vi "SerialComMain.vi"() -> ()   [LabVIEW 2021]
uses:
  MainDataTypedef.ctl
  <vilib>/Instr/_visa.llb/VISA Configure Serial Port (Instr).vi
panel:
  out "bytes read":u32
  out "NowTime":timestamp
  in  "ClosePort":bool
  in  "OpenProt":bool
  in  "flow control":u16(ring) items=["None"=0, "XON/XOFF"=1, "RTS/CTS"=2, "DTR/DSR"=4]
  in  "stop bits":u16(ring)=10 items=["1.0"=10, "1.5"=15, "2.0"=20]
  in  "parity":u16(ring) items=["None", "Odd", "Even", "Mark", "Space"]
  in  "data bits":u16=8 min=5 max=8 step=1
  in  "baud rate":u32=9600
  in  "delay before read (ms)":u32=500
  in  "VISA resource name":refnum<visa-resource-name>="COM1"
  out "Response":string
  in  "Command":string="*IDN?\n"
  in  "SerialSend":bool
  out "MsgString":string
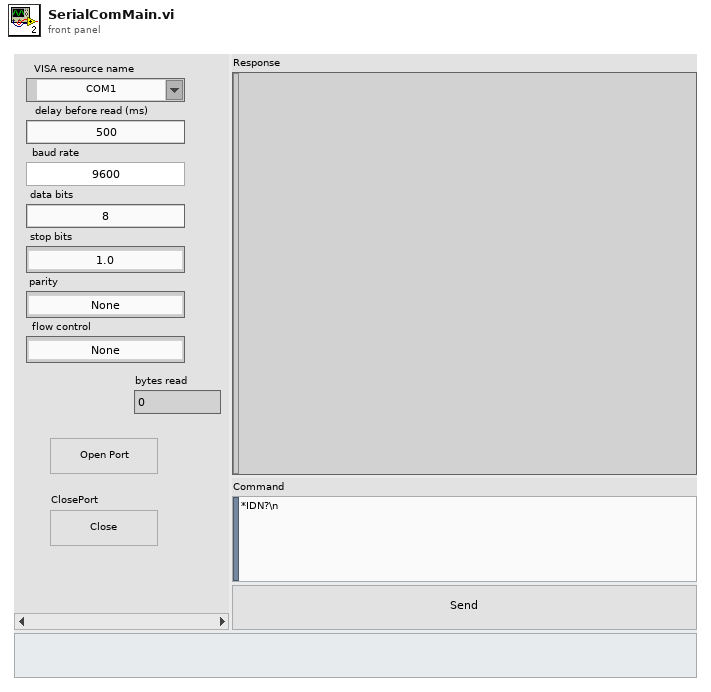
[diagram p1: front panel]
types:
  T1 = typedef "MainDataTypedef.ctl" = cluster{"NowTime":timestamp, "MsgString":string, "VISAResource":refnum<visa-resource-name>, "BytesRead":u32, "Respones":string, "PortOpen?":bool}
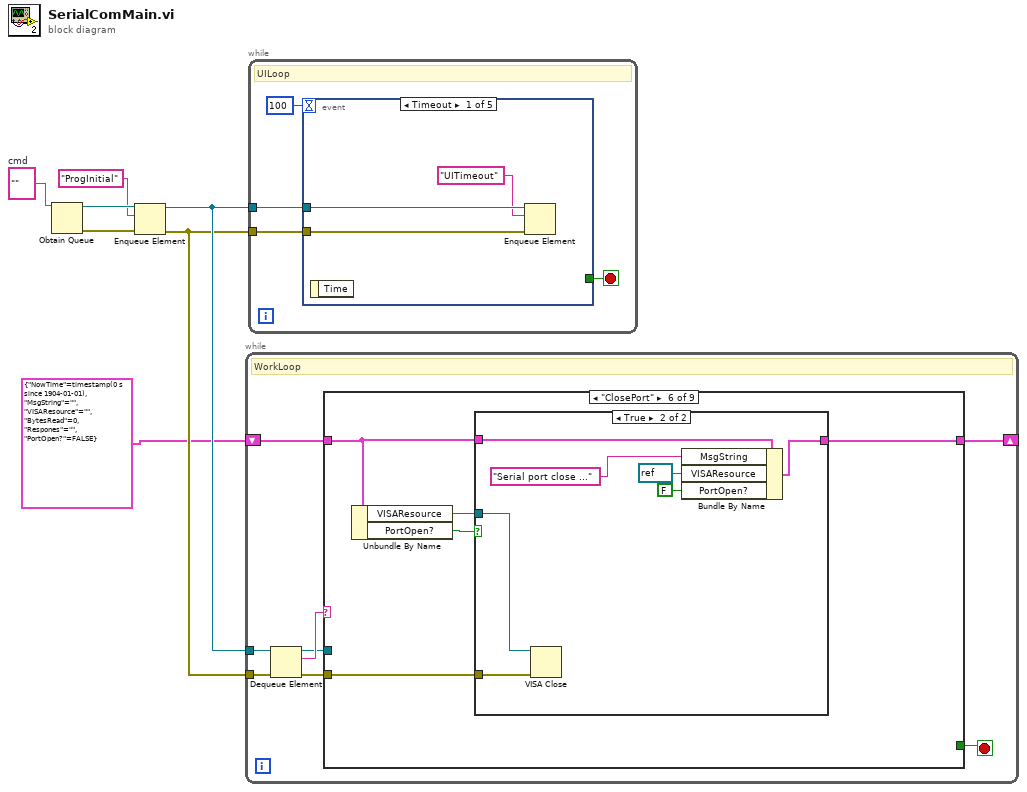
[diagram p0: block diagram]
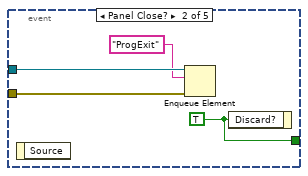
[diagram p2: hidden frame]
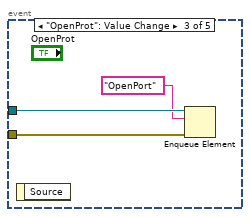
[diagram p3: hidden frame]
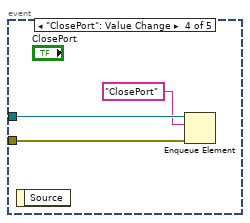
[diagram p4: hidden frame]
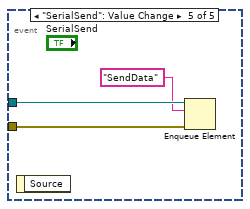
[diagram p5: hidden frame]
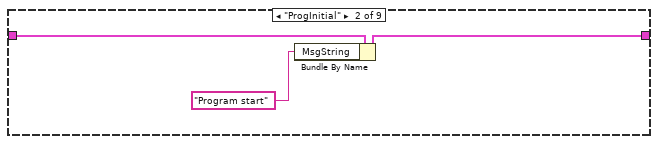
[diagram p7: hidden frame]
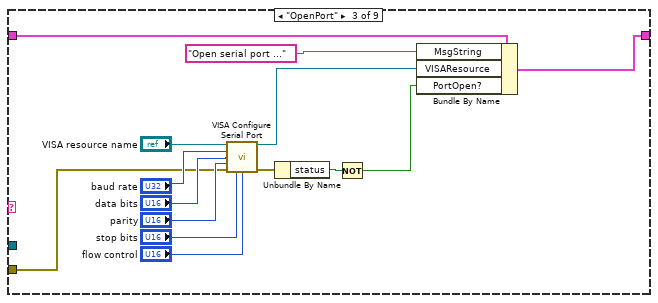
[diagram p8: hidden frame]
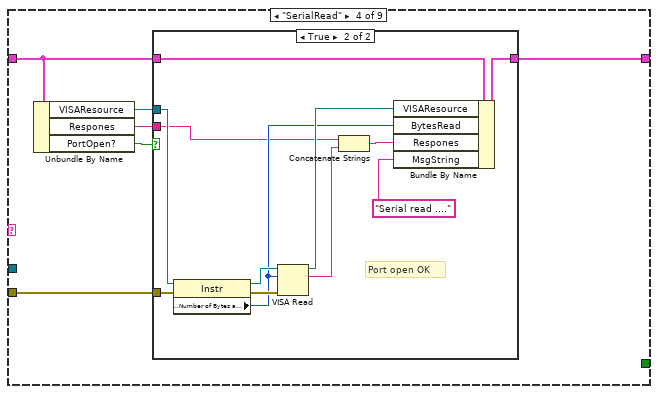
[diagram p9: hidden frame]
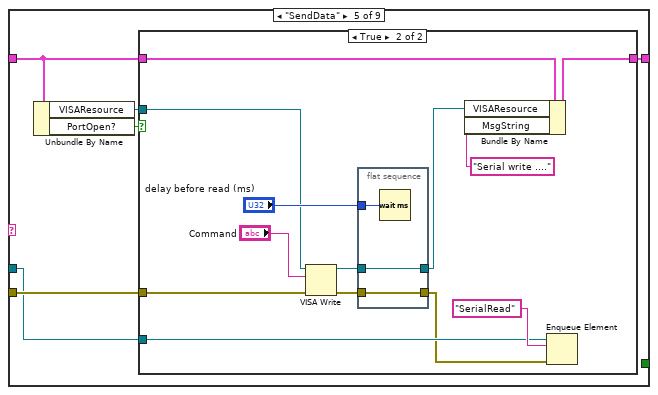
[diagram p11: hidden frame]
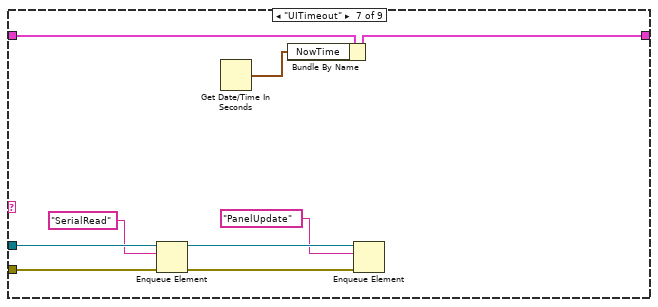
[diagram p14: hidden frame]
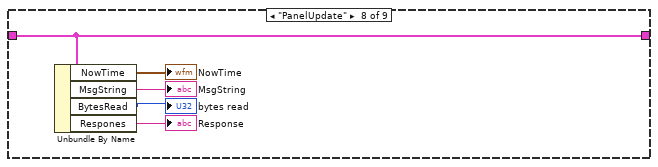
[diagram p15: hidden frame]
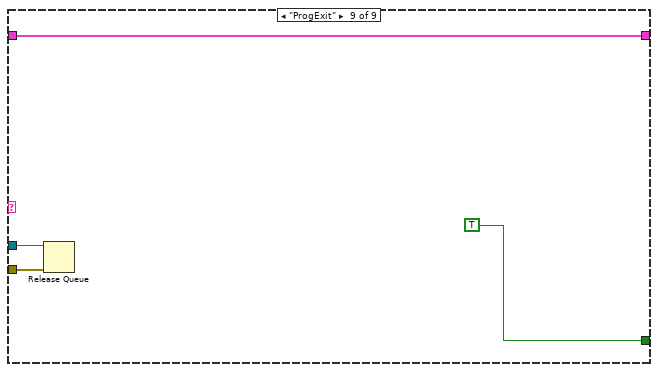
[diagram p16: hidden frame]
diagram:
  w5 = ""  # cmd
  n1 = Obtain Queue(element data type=w5) -> (queue out=w7:refnum<queue>, error out=w6:errorcluster)  [unwired: 4 in, 1 out]
  n2 = Enqueue Element(queue=w7, element="ProgInitial", error in (no error)=w6) -> (queue out=w3:refnum<queue>, error out=w2:errorcluster)  [unwired: 1 in, 1 out]
  n3 = while {
    tunnel: w3 -> [w15]
    tunnel: w2 -> [w14]
    shift-right: [w12] -> _
    shift-left: T1 {"NowTime"=timestamp(0 s since 1904-01-01), "MsgString"="", "VISAResource"="", "BytesRead"=0, "Respones"="", "PortOpen?"=FALSE} -> [w11]
    stop <- w8 stop-if-true
    # "WorkLoop"
    n4 = Dequeue Element(queue=w15, error in (no error)=w14) -> (queue out=w10:refnum<queue>, element=w13:string, error out=w9:errorcluster)  [unwired: 1 in, 1 out]
    n5 = case shown="\"ClosePort\"" w13 {
      tunnel: [w16 w18 w32 w36 w55 w80 w96 w102 w106] -> w12
      tunnel: w11 -> [w16 w19 w33 w39 w58 w79 w97 w102 w106]
      tunnel: w10 -> [_ _ _ _ w53 _ w94 _ w105]
      tunnel: w9 -> [_ _ w24 w37 w56 w77 w93 _ w104]
      tunnel: [_ _ _ _ _ _ _ _ TRUE ("Discard?")] -> w8
      frame Default {
      }
      frame "ProgInitial" {
        n6 = Bundle By Name(cluster=w19, "MsgString"="Program start" ("message")) -> (w18:T1)
      }
      frame "OpenPort" {
        n7 = call-poly "VISA Configure Serial Port"("VISA resource name"="VISA resource name", "baud rate (9600)"="baud rate", "data bits (8)"="data bits", "parity (0:none)"="parity", "error in (no error)"=w24, "stop bits (10: 1 bit)"="stop bits", "flow control (0:none)"="flow control") -> ("VISA resource name out"=w23:refnum<visa-resource-name>, "error out"=w22:errorcluster)  [unwired: 2 in, 5 out]
        n8 = Unbundle By Name(w22) -> ("status"=w21:bool)
        n9 = Not(x=w21) -> (.not. x?=w20:bool)
        n10 = Bundle By Name(cluster=w33, "MsgString"="Open serial port ..." ("message"), "VISAResource"=w23, "PortOpen?"=w20) -> (w32:T1)
      }
      frame "SerialRead" {
        n11 = Unbundle By Name(w39) -> ("VISAResource"=w38:refnum<visa-resource-name>, "Respones"=w35:string, "PortOpen?"=w34:bool)
        n12 = case shown="True" w34 {
          tunnel: w39 -> [w40 w50]
          tunnel: w38 -> [_ w49]
          tunnel: w37 -> [_ w48]
          tunnel: [w40 w47] -> w36
          tunnel: w35 -> [_ w42]
          frame False {
            # "Port not open"
          }
          frame True {
            # "Port open OK"
            n13 = property class="Instr"(reference=w49, error in=w48) -> (reference out=w51:refnum<visa-resource-name>, error out=w52:errorcluster, "Serial Settings:Number of Bytes at Serial Port"=w45:u32)
            n14 = VISA Read(VISA resource name=w51, byte count=w45, error in (no error)=w52) -> (VISA resource name out=w46:refnum<visa-resource-name>, read buffer=w44:string)  [unwired: 2 out]
            n15 = Concatenate Strings(w42, w44) -> (w43:string)
            n16 = Bundle By Name(cluster=w50, "VISAResource"=w46, "BytesRead"=w45, "Respones"=w43, "MsgString"="Serial read ....") -> (w47:T1)
          }
        }
      }
      frame "SendData" {
        n17 = Unbundle By Name(w58) -> ("VISAResource"=w57:refnum<visa-resource-name>, "PortOpen?"=w54:bool)
        n18 = case shown="True" w54 {
          tunnel: w58 -> [w59 w72]
          tunnel: w57 -> [_ w65]
          tunnel: w56 -> [_ w63]
          tunnel: [w59 w71] -> w55
          tunnel: w53 -> [_ w61]
          frame False {
            # "Port not open"
          }
          frame True {
            n19 = VISA Write(VISA resource name=w65, write buffer="Command", error in (no error)=w63) -> (VISA resource name out=w67:refnum<visa-resource-name>, error out=w66:errorcluster)  [unwired: 1 out]
            n20 = flat-sequence {
              tunnel: w66 -> [w74]
              tunnel: [w74] -> w60
              tunnel: w67 -> [w73]
              tunnel: [w73] -> w64
              tunnel: "delay before read (ms)" -> [w75]
              frame #0 {
                n21 = Wait (ms)(milliseconds to wait=w75) -> ()  [unwired: 1 out]
              }
            }
            n22 = Bundle By Name(cluster=w72, "VISAResource"=w64, "MsgString"="Serial write ....") -> (w71:T1)
            n23 = Enqueue Element(queue=w61, element="SerialRead", error in (no error)=w60) -> ()  [unwired: 1 in, 3 out]
          }
        }
      }
      frame "ClosePort" {
        n24 = Unbundle By Name(w79) -> ("VISAResource"=w78:refnum<visa-resource-name>, "PortOpen?"=w76:bool)
        n25 = case shown="True" w76 {
          tunnel: [w81 w88] -> w80
          tunnel: w79 -> [w81 w86]
          tunnel: w78 -> [_ w85]
          tunnel: w77 -> [_ w84]
          frame False {
            # "port not open"
          }
          frame True {
            n26 = VISA Close(VISA resource name=w85, error in (no error)=w84) -> ()  [unwired: 1 out]
            n27 = Bundle By Name(cluster=w86, "MsgString"="Serial port close ..." ("message"), "VISAResource"=refnum<visa-resource-name> refnum, "PortOpen?"=FALSE) -> (w88:T1)
          }
        }
      }
      frame "UITimeout" {
        n28 = Enqueue Element(queue=w94, element="SerialRead", error in (no error)=w93) -> (queue out=w92:refnum<queue>, error out=w91:errorcluster)  [unwired: 1 in, 1 out]
        n29 = Get Date/Time In Seconds() -> (seconds since 1Jan1904=w95:timestamp)
        n30 = Bundle By Name(cluster=w97, "NowTime"=w95) -> (w96:T1)
        n31 = Enqueue Element(queue=w92, element="PanelUpdate", error in (no error)=w91) -> ()  [unwired: 1 in, 3 out]
      }
      frame "PanelUpdate" {
        n32 = Unbundle By Name(w102) -> ("NowTime"=→"NowTime":timestamp, "MsgString"=→"MsgString":string, "BytesRead"=→"bytes read":u32, "Respones"=→"Response":string)
      }
      frame "ProgExit" {
        n33 = Release Queue(queue=w105, error in (no error)=w104) -> ()  [unwired: 1 in, 3 out]
      }
    }
  }
  n34 = while {
    tunnel: w3 -> [w109]
    tunnel: w2 -> [w108]
    stop <- w107 stop-if-true
    # "UILoop"
    n35 = event shown="[0] Timeout" {
      selector: _ -> [_ _ _ _ _]
      dyn-events: _ -> [_ _ _ _ _]
      timeout: 100 -> [_ _ _ _ _]
      tunnel: w109 -> [w113 w117 w120 w123 w126]
      tunnel: w108 -> [w112 w116 w119 w122 w125]
      tunnel: [_ w115 _ _ _] -> w107
      event Timeout {
        n36 = event-data() -> ()  [unwired: 1 in, 1 out]
        n37 = Enqueue Element(queue=w113, element="UITimeout", error in (no error)=w112) -> ()  [unwired: 1 in, 3 out]
      }
      event Panel Close? {
        w115 = TRUE ("Discard?")
        n38 = event-data() -> ()  [unwired: 1 in, 1 out]
        n39 = Enqueue Element(queue=w117, element="ProgExit", error in (no error)=w116) -> ()  [unwired: 1 in, 3 out]
        n40 = event-data("Discard?"=w115) -> ()  [unwired: 1 in, 1 out]
      }
      event "OpenProt": Value Change {
        n41 = event-data() -> ()  [unwired: 1 in, 1 out]
        n42 = Enqueue Element(queue=w120, element="OpenPort", error in (no error)=w119) -> ()  [unwired: 1 in, 3 out]
      }
      event "ClosePort": Value Change {
        n43 = event-data() -> ()  [unwired: 1 in, 1 out]
        n44 = Enqueue Element(queue=w123, element="ClosePort", error in (no error)=w122) -> ()  [unwired: 1 in, 3 out]
      }
      event "SerialSend": Value Change {
        n45 = event-data() -> ()  [unwired: 1 in, 1 out]
        n46 = Enqueue Element(queue=w126, element="SendData", error in (no error)=w125) -> ()  [unwired: 1 in, 3 out]
      }
    }
  }
